vi "DetectPCIDGs.vi"(8 "error in (no error)":errorcluster, 11 "BME_DG_System in":refnum<class "BME_DG_System.lvclass">) -> (0 "error out":errorcluster, 1 "Errors":errorcluster[](array[cluster]), 2 "InstalledDGs":T1[](array[typedef]), 3 "BME_DG_System out":refnum<class "BME_DG_System.lvclass">, 5 "#DGs":i32)   [LabVIEW 2009, in "POLARIS BME DG.lvlib" / "BME_DG_System.lvclass"]
uses:
  BME_DG_System.lvclass
  DetectDG.ctl
  <vilib>/Utility/miscctls.llb/LVStringsAndValuesArrayTypeDef.ctl
  POLARIS BME DG.lvlib
panel:
  in  "?":T1
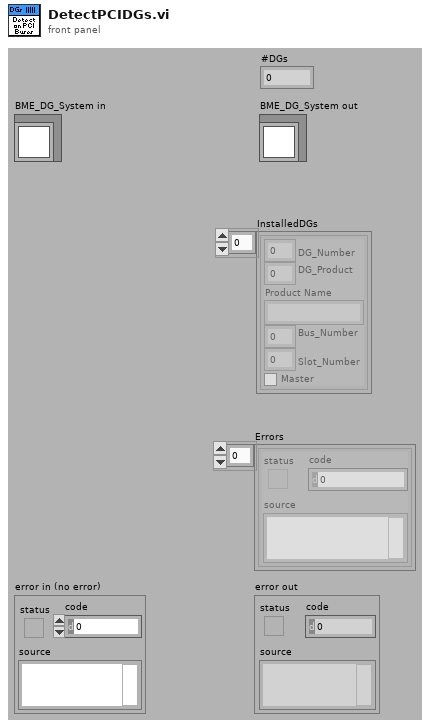
[diagram p1: front panel]
types:
  T1 = typedef "POLARIS BME DG.lvlib/DetectDG.ctl" = cluster{"DG_Number":i32, "DG_Product":i32, "Product Name":string, "Bus_Number":i32, "Slot_Number":i32, "Master":bool}
  T2 = typedef "LVStringsAndValuesArrayTypeDef.ctl" = cluster{"String":string, "Value":ext}[]
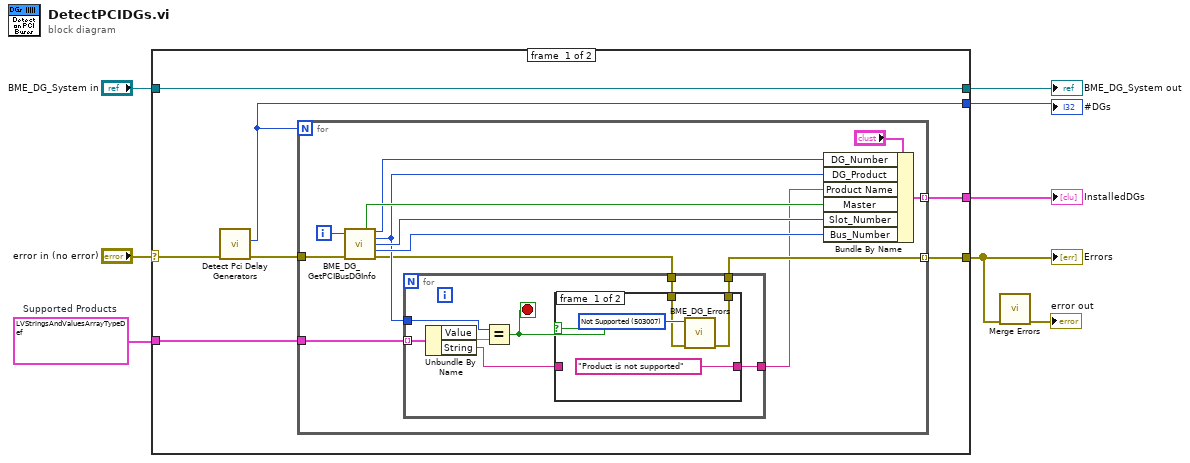
[diagram p0: block diagram]
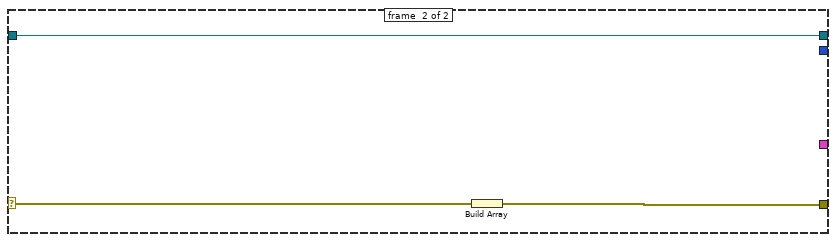
[diagram p3: hidden frame]
diagram:
  w4 = T2 [{"String"="SRS_DG135", "Value"=1.0}, {"String"="BME_DP01", "Value"=2.0}, {"String"="BME_G02V3", "Value"=3.0}, {"String"="BME_SG02V4", "Value"=4.0}, {"String"="BME_G04", "Value"=5.0}, {"String"="BME_G02V1", "Value"=6.0}, {"String"="BME_G02V2", "Value"=7.0}, {"String"="BME_SG02V1", "Value"=8.0}, {"String"="BME_SG02V2", "Value"=9.0}, {"String"="BME_SG02V3", "Value"=10.0}, {"String"="BME_G03V1", "Value"=11.0}, {"String"="BME_G03V2", "Value"=12.0}, {"String"="BME_SG02V5", "Value"=13.0}, {"String"="BME_G03V3", "Value"=14.0}, {"String"="BME_G03V4", "Value"=15.0}, {"String"="BME_SG02V6", "Value"=16.0}, {"String"="BME_G03V5", "Value"=17.0}, {"String"="BME_G05V1", "Value"=18.0}, {"String"="BME_G05V2", "Value"=19.0}, {"String"="BME_G05V3", "Value"=20.0}, {"String"="BME_SG02V7", "Value"=21.0}, {"String"="BME_SG02P1", "Value"=31.0}, {"String"="BME_G03P1", "Value"=32.0}, {"String"="BME_G05P1", "Value"=33.0}, {"String"="BME_SG02P2", "Value"=34.0}, {"String"="BME_G03P2", "Value"=35.0}, {"String"="BME_SG02P3", "Value"=36.0}, {"String"="BME_SG05P1", "Value"=37.0}, {"String"="BME_G05P2", "Value"=38.0}, {"String"="BME_SG05P2", "Value"=39.0}, {"String"="BME_G05P3", "Value"=40.0}, {"String"="BME_SG02P4", "Value"=41.0}, {"String"="BME_SG02P5", "Value"=42.0}, {"String"="BME_SG05P3", "Value"=43.0}, {"String"="BME_SG08P1", "Value"=44.0}, {"String"="BME_SG08P2", "Value"=45.0}]  # Supported Products
  n1 = case shown="No Error" "error in (no error)" {
    selector: "error in (no error)" -> [w14 w45]
    tunnel: [w11 w43] -> w3
    tunnel: [w15 w44] -> w6
    tunnel: "BME_DG_System in" -> [w15 w44]
    tunnel: w4 -> [w12 _]
    tunnel: [w10 _] -> w5
    tunnel: [w9 _] -> w1
    frame #0 {
      n2 = call "Detect Pci Delay Generators.vi"("error in (no error)"=w14) -> ("error out"=w13:errorcluster, "Number of Generators"=w9:i32)  [unwired: 8 in, 1 out]
      n3 = for {
        N: w9 -> [_]
        tunnel: w12 -> [w22]
        tunnel: w13 -> [w27]
        tunnel: [w19] -> w11 mode=indexing
        tunnel: [w16] -> w10 mode=indexing
        i -> [w28]
        n4 = call "BME_DG_GetPCIBusDGInfo.vi"("DG_Number in"=w28, "error in (no error)"=w27) -> ("Master"=w26:bool, "DG_Number out"=w25:i32, "DG_Product"=w21:i32, "SlotNumber"=w24:i32, "Bus_Number"=w23:i32, "error out"=w20:errorcluster)  [unwired: 8 in]
        n5 = for {
          tunnel: w22 -> [w36] mode=indexing
          tunnel: w21 -> [w34]
          tunnel: w20 -> [w32]
          tunnel: [w31] -> w19
          tunnel: [w30] -> w18
          stop <- w33 stop-if-true
          n6 = Unbundle By Name(w36) -> ("Value"=w35:ext, "String"=w29:string)
          n7 = Equal?(x=w34, y=w35) -> (x = y?=w33:bool)
          n8 = case shown="False" w33 {
            tunnel: w32 -> [w39 w42]
            tunnel: [w38 w42] -> w31
            tunnel: ["Product is not supported" ("f") w41] -> w30
            tunnel: w29 -> [_ w41]
            frame #0 {
              w40 = 503007 items=["Channel refers itself"=503001, "Deadloop"=503002, "Negative Delay"=503003, "Delay Card not found"=503004, "Channel not found"=503005, "Parse Error"=503006, "Not Supported"=503007] ("error")
              n9 = call "BME_DG_Errors.vi"("error in (no error)"=w39, "error"=w40) -> ("error out"=w38:errorcluster)  [unwired: 9 in]
            }
            frame #1 {
            }
          }
        }
        n10 = Bundle By Name(cluster="?", "DG_Number"=w25, "DG_Product"=w21, "Product Name"=w18, "Master"=w26, "Slot_Number"=w24, "Bus_Number"=w23) -> (w16:T1)
      }
    }
    frame #1 {
      n11 = Build Array(w45) -> (w43:errorcluster[])
    }
  }
  "BME_DG_System out" <- w6
  "Errors" <- w3
  "InstalledDGs" <- w5
  "#DGs" <- w1
  n12 = call <vilib>:"Merge Errors.vi"("error array in"=w3) -> ("error out"=→"error out":errorcluster)  [unwired: 6 in]
